vi "StringTocommand.vi"(8 "error in":errorcluster, 11 "data string":string) -> (0 "error out":errorcluster, 1 "output cluster":T1, 2 "Error?":bool, 3 "Data out":string, 10 "data":string)   [LabVIEW 2016]
doc: "Parses input string to command (using the typedef'd command enum) and data. command and data are separated using whitespace."
uses:
  DataType.ctl
  data_command_enum.ctl
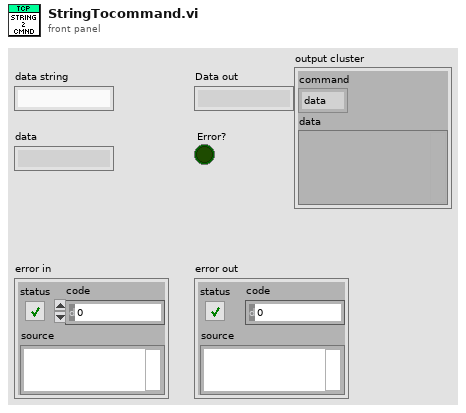
[diagram p1: front panel]
types:
  T1 = typedef "DataType.ctl" = cluster{"command":T2, "data":variant}
  T2 = typedef "data_command_enum.ctl" = enum16{"data", "display", "quit", "save", "filepath", "weak left", "state", "weak right", "strong left", "strong right", "stopRecording", "close", "sid"}
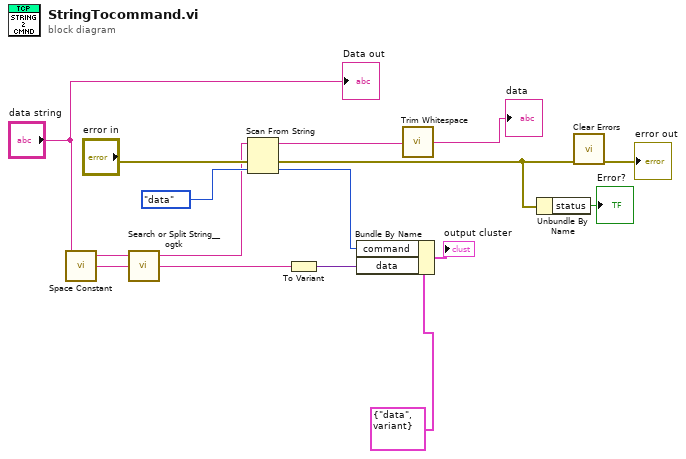
[diagram p0: block diagram]
diagram:
  n1 = call <vilib>:"Space Constant.vi"() -> ("String"=w3:string)
  n2 = call <userlib>:"Search or Split String__ogtk.vi"("search string/char (-)"=w3, "string"="data string") -> ("substring after match"=w2:string, "substring before match"=w4:string)  [unwired: 1 in, 1 out]
  n3 = Scan From String(input string=w4, error in="error in", default 1=data_command_enum."data" ("command")) -> (remaining string=w14:string, error out=w11:errorcluster, output 1=w15:T2)  [unwired: 2 in, 1 out]
  n4 = To Variant(anything=w2) -> (Variant=w1:variant)
  n5 = Bundle By Name(cluster=T1 {"command"=enum."data", "data"=variant} ("Cluster"), "command"=w15, "data"=w1) -> (→"output cluster":T1)
  n6 = call <vilib>:"Trim Whitespace.vi"("string"=w14) -> ("trimmed string"=→"data":string)  [unwired: 1 in]
  n7 = Unbundle By Name(w11) -> ("status"=→"Error?":bool)
  n8 = call <vilib>:"Clear Errors.vi"("error in (no error)"=w11) -> ("error out"=→"error out":errorcluster)  [unwired: 5 in, 1 out]
  "Data out" <- "data string"
